vi "Extended Power Spectra.vi"(6 "Normalize?":bool, 8 "Error In":errorcluster, 9 "Waveforms In":waveform(dbl)[](array[waveform]), 10 "Upsampling pow. of 2":dbl=4.0 format="%#_13g") -> (0 "Error Out":errorcluster, 1 "Power Spectra":cluster{"f0":dbl, "df":dbl, "Magnitude":dbl[]}[](array[cluster]))   [LabVIEW 2019]
uses:
  <vilib>/Analysis/4window.llb/windowTd.ctl
  <vilib>/measure/maspectr.llb/Power Spectrum and PSD Export Mode.ctl
  <vilib>/measure/maspectr.llb/FFT Power Spectrum and PSD for N Chan.vi
  <vilib>/measure/NI_MAPro.lvlib
  <vilib>/Analysis/NI_AALPro.lvlib
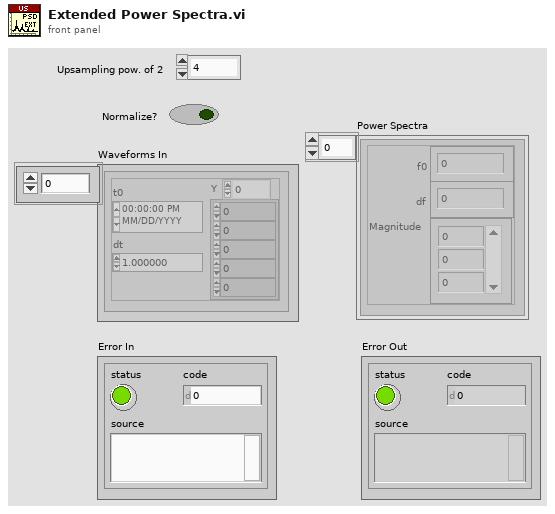
[diagram p1: front panel]
types:
  T1 = typedef "NI_MAPro.lvlib/Power Spectrum and PSD Export Mode.ctl" = u16
  T2 = typedef "NI_AALPro.lvlib/windowTd.ctl" = u32
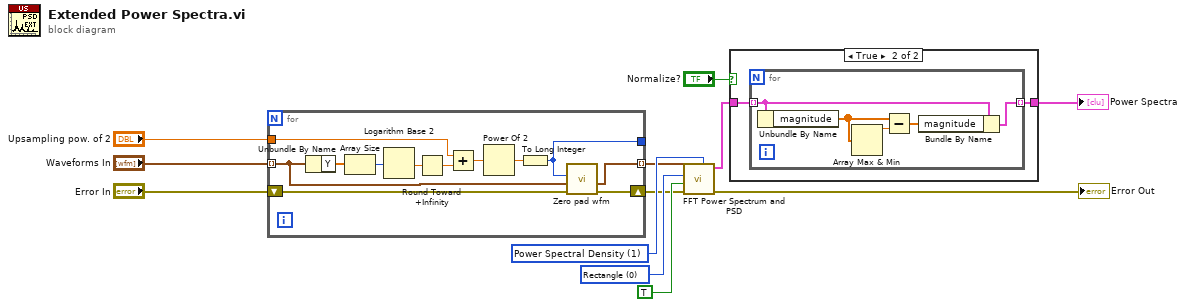
[diagram p0: block diagram]
diagram:
  w6 = T1 1 items=["Power Spectrum", "Power Spectral Density"] ("export mode")
  w7 = T2 0 items=["Rectangle"=0, "Hanning"=1, "Hamming"=2, "Blackman-Harris"=3, "Exact Blackman"=4, "Blackman"=5, "Flat Top"=6, "4 Term B-Harris "=7, "7 Term B-Harris"=8, "Low Sidelobe"=9, "Blackman Nuttall"=11, "Triangle"=30, "Bartlett-Hanning"=31, "Bohman"=32, "Parzen"=33, "Welch"=34, "Kaiser"=60, "Dolph-Chebyshev"=61, "Gaussian"=62] ("window")
  n1 = for {
    tunnel: "Upsampling pow. of 2" -> [w21]
    tunnel: [w17] -> _
    shift-right: [w16] -> w3
    shift-left: "Error In" -> [w13]
    tunnel: "Waveforms In" -> [w15] mode=indexing
    tunnel: [w14] -> w2 mode=indexing
    n2 = Unbundle By Name(w15) -> ("Y"=w20:dbl[])
    n3 = Array Size(array=w20) -> (size(s)=w24:i32)
    n4 = Logarithm Base 2(1:w24) -> (0:w18:dbl)
    n5 = Round Toward +Infinity(x=w18) -> (ceil(x): smallest int >= x=w22:dbl)
    n6 = Add(x=w21, y=w22) -> (x+y=w23:dbl)
    n7 = Power Of 2(x=w23) -> (2^x=w19:dbl)
    n8 = To Long Integer(number=w19) -> (32bit integer=w17:i32)
    n9 = call "Zero pad wfm.vi"("Error In"=w13, "Waveform In"=w15, "New size"=w17) -> ("Error Out"=w16:errorcluster, "Zero padded waveform"=w14:waveform(dbl))  [unwired: 7 in]
  }
  n10 = call-poly <vilib>:"FFT Power Spectrum and PSD.vi"("export mode"=w6, "error in (no error)"=w3, "dB On (F)"=TRUE, "window"=w7, "time signals"=w2) -> ("error out"=→"Error Out":errorcluster, "Power Spectrum / PSD"=w4:cluster{"f0":dbl, "df":dbl, "magnitude":dbl[]}[])  [unwired: 3 in, 2 out]
  n11 = case shown="True" "Normalize?" {
    tunnel: w4 -> [w25 w27]
    tunnel: [w25 w26] -> w9
    frame False {
    }
    frame True {
      n12 = for {
        tunnel: w27 -> [w29] mode=indexing
        tunnel: [w28] -> w26 mode=indexing
        n13 = Unbundle By Name(w29) -> ("magnitude"=w31:dbl[])
        n14 = Array Max & Min(array=w31) -> (max value=w32:dbl)  [unwired: 3 out]
        n15 = Subtract(x=w31, y=w32) -> (x-y=w30:dbl[])
        n16 = Bundle By Name(cluster=w29, "magnitude"=w30) -> (w28:cluster{"f0":dbl, "df":dbl, "magnitude":dbl[]})
      }
    }
  }
  "Power Spectra" <- w9
